vi "shared memory read.vi"(6 "channel classification":T1, 8 "error in":errorcluster, 10 "data table":T2, 11 "module in":refnum<class "Shared Memory Runtime.lvclass">) -> (0 "error out":errorcluster, 2 "data table out":T2, 3 "module out":refnum<class "Shared Memory Runtime.lvclass">)   [LabVIEW 2013, in "Shared Memory Runtime.lvclass"]
uses:
  Shared Memory Runtime.lvclass
  <vilib>/NI/Tag Bus/table/data table.ctl
  <vilib>/NI/Tag Bus Module Framework/channel/channel classification.ctl
  <vilib>/NI/Tag Bus/table/data polymorphs/write many/write Doubles.vi
  <vilib>/NI/Tag Bus/table/data polymorphs/write many/write Singles.vi
  <vilib>/NI/Tag Bus/table/data polymorphs/write many/write I64s.vi
  <vilib>/NI/Tag Bus/table/data polymorphs/write many/write I32s.vi
  <vilib>/NI/Tag Bus/table/data polymorphs/write many/write I16s.vi
  <vilib>/NI/Tag Bus/table/data polymorphs/write many/write I8s.vi
  <vilib>/NI/Tag Bus/table/data polymorphs/write many/write U64s.vi
  <vilib>/NI/Tag Bus/table/data polymorphs/write many/write U32s.vi
  <vilib>/NI/Tag Bus/table/data polymorphs/write many/write U16s.vi
  <vilib>/NI/Tag Bus/table/data polymorphs/write many/write U8s.vi
  <vilib>/NI/Tag Bus/table/data polymorphs/write many/write Booleans.vi
  <vilib>/National Instruments/Shared Memory Library for Linux RT/VIs/Miscellaneous/Get Shared Object Path.vi
  <vilib>/Utility/libraryn.llb/Check if File or Folder Exists.vi
  <vilib>/Utility/error.llb/Error Cluster From Error Code.vi
  <vilib>/NI/Tag Bus/table/data table.lvlib
  <vilib>/National Instruments/Shared Memory Library for Linux RT/Shared Memory.lvlib
  <vilib>/NI/Tag Bus Module Framework/channel/TBM channel.lvclass
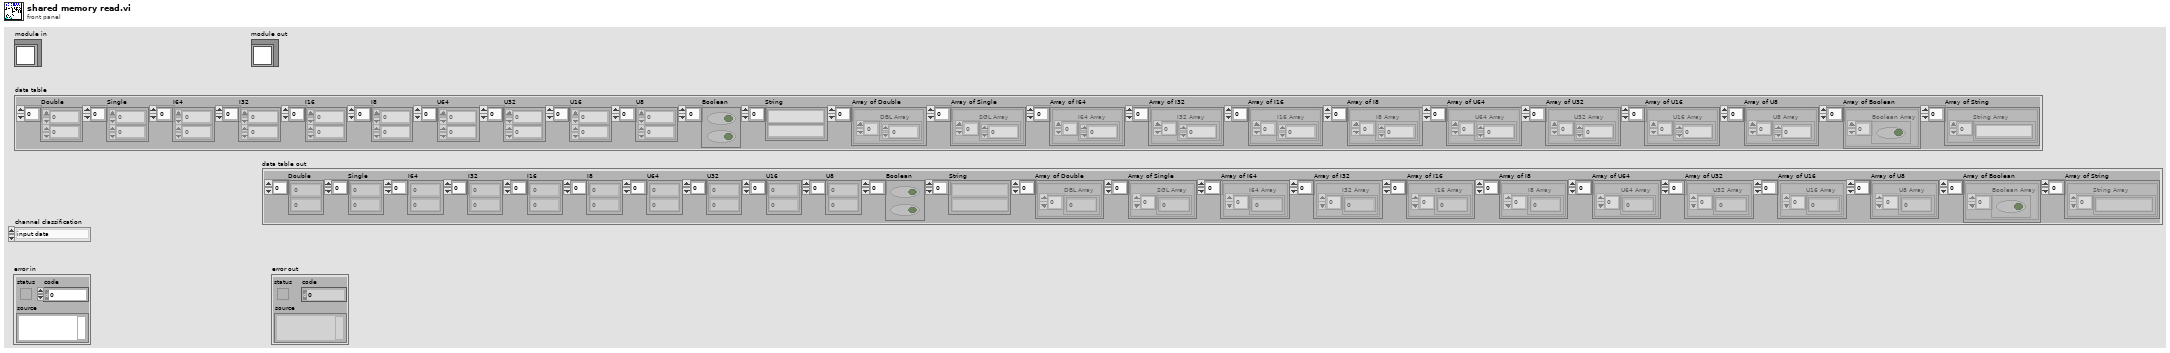
[diagram p1: front panel]
types:
  T1 = typedef "TBM channel.lvclass/channel classification.ctl" = enum16{"input data", "output data", "processing parameter", "processing result"}
  T2 = typedef "tag bus.lvlib/data table.lvlib/data table.ctl" = cluster{"Double":dbl[], "Single":sgl[], "I64":i64[], "I32":i32[], "I16":i16[], "I8":i8[], "U64":u64[], "U32":u32[], "U16":u16[], "U8":u8[], "Boolean":bool[], "String":string[], "Array of Double":cluster{"DBL Array":dbl[]}[], "Array of Single":cluster{"SGL Array":sgl[]}[], "Array of I64":cluster{"I64 Array":i64[]}[], "Array of I32":cluster{"I32 Array":i32[]}[], "Array of I16":cluster{"I16 Array":i16[]}[], "Array of I8":cluster{"I8 Array":i8[]}[], "Array of U64":cluster{"U64 Array":u64[]}[], "Array of U32":cluster{"U32 Array":u32[]}[], "Array of U16":cluster{"U16 Array":u16[]}[], "Array of U8":cluster{"U8 Array":u8[]}[], "Array of Boolean":cluster{"Boolean Array":bool[]}[], "Array of String":cluster{"String Array":string[]}[]}
  T3 = typedef "shared memory runtime.lvclass/shared memory module runtime.ctl" = cluster{"channel classification":T1, "data type":T4, "pointer to shared memory":u64, "number of elements":u64, "data dictionary index":cluster{i32[]}, "shared memory":T5}
  T4 = typedef "tag bus.lvlib/tag descriptor.lvclass/Data Type.ctl" = enum16{"Double", "Single", "I64", "I32", "I16", "I8", "U64", "U32", "U16", "U8", "Boolean", "String", "Array of Double", "Array of Single", "Array of I64", "Array of I32", "Array of I16", "Array of I8", "Array of U64", "Array of U32", "Array of U16", "Array of U8", "Array of Boolean", "Array of String"}
  T5 = typedef "Shared Memory Class Reference.ctl" = refnum<data-value>
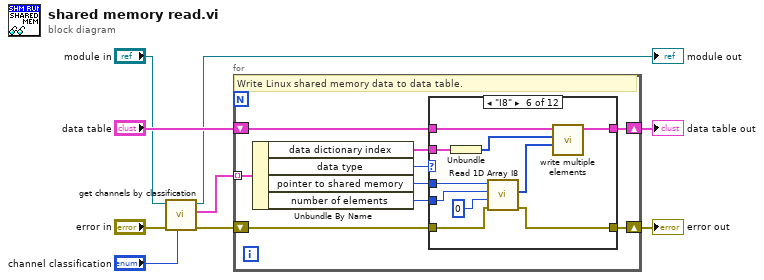
[diagram p0: block diagram]
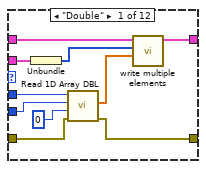
[diagram p2: hidden frame]
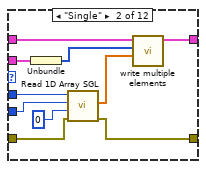
[diagram p3: hidden frame]
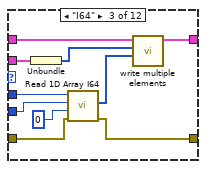
[diagram p4: hidden frame]
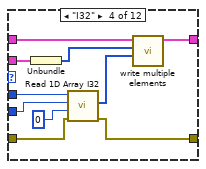
[diagram p5: hidden frame]
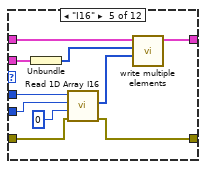
[diagram p6: hidden frame]
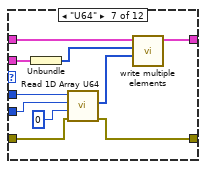
[diagram p7: hidden frame]
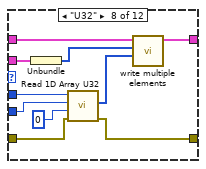
[diagram p8: hidden frame]
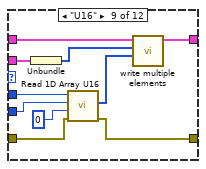
[diagram p9: hidden frame]
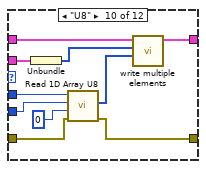
[diagram p10: hidden frame]
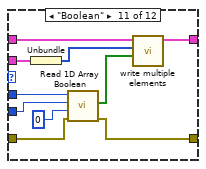
[diagram p11: hidden frame]
diagram:
  n1 = call "get channels by classification.vi"("channel classification"="channel classification", "error in"="error in", "shared memory runtime in"="module in") -> ("error out"=w1:errorcluster, "channels"=w4:T3[], "shared memory runtime out"=→"module out":refnum<class "Shared Memory Runtime.lvclass">)  [unwired: 6 in]
  n2 = for {
    tunnel: w4 -> [w16] mode=indexing
    shift-right: [w11] -> w7
    shift-left: w1 -> [w12]
    shift-right: [w18] -> w8
    shift-left: "data table" -> [w17]
    # "Write Linux shared memory data to data table."
    n3 = Unbundle By Name(w16) -> ("data dictionary index"=w10:cluster{i32[]}, "data type"=w13:T4, "pointer to shared memory"=w15:u64, "number of elements"=w14:u64)
    n4 = case shown="\"I8\"" w13 {
      tunnel: w17 -> [w28 w38 w48 w58 w68 w78 w88 w98 w108 w118 w128 w130]
      tunnel: [w27 w37 w47 w57 w67 w77 w87 w97 w107 w117 w127 w130] -> w18
      tunnel: w12 -> [w20 w30 w40 w50 w60 w70 w80 w90 w100 w110 w121 w129]
      tunnel: [w19 w29 w39 w49 w59 w69 w79 w89 w99 w109 w120 w129] -> w11
      tunnel: w15 -> [w22 w32 w42 w52 w62 w72 w82 w92 w102 w112 w123 _]
      tunnel: w14 -> [w21 w31 w41 w51 w61 w71 w81 w91 w101 w111 w122 _]
      tunnel: w10 -> [w26 w36 w46 w56 w66 w76 w86 w96 w106 w116 w126 _]
      frame "Double" {
        n5 = Unbundle(w26) -> (w25:i32[])
        n6 = call <vilib>:"Read 1D Array DBL.vi"("error in (no error)"=w20, "start index"=u64 0, "number of elements"=w21, "pointer"=w22) -> ("error out"=w19:errorcluster, "value"=w23:dbl[])  [unwired: 5 in, 1 out]
        n7 = call-poly <vilib>:"write multiple elements.vi"("values"=w23, "indices"=w25, "data table in"=w28) -> ("data table out"=w27:T2)  [unwired: 8 in]
      }
      frame "Single" {
        n8 = Unbundle(w36) -> (w35:i32[])
        n9 = call <vilib>:"Read 1D Array SGL.vi"("error in (no error)"=w30, "start index"=u64 0, "number of elements"=w31, "pointer"=w32) -> ("error out"=w29:errorcluster, "value"=w33:sgl[])  [unwired: 5 in, 1 out]
        n10 = call-poly <vilib>:"write multiple elements.vi"("values"=w33, "indices"=w35, "data table in"=w38) -> ("data table out"=w37:T2)  [unwired: 8 in]
      }
      frame "I64" {
        n11 = Unbundle(w46) -> (w45:i32[])
        n12 = call <vilib>:"Read 1D Array I64.vi"("error in (no error)"=w40, "start index"=u64 0, "number of elements"=w41, "pointer"=w42) -> ("error out"=w39:errorcluster, "value"=w43:i64[])  [unwired: 5 in, 1 out]
        n13 = call-poly <vilib>:"write multiple elements.vi"("values"=w43, "indices"=w45, "data table in"=w48) -> ("data table out"=w47:T2)  [unwired: 8 in]
      }
      frame "I32" {
        n14 = Unbundle(w56) -> (w55:i32[])
        n15 = call <vilib>:"Read 1D Array I32.vi"("error in (no error)"=w50, "start index"=u64 0, "number of elements"=w51, "pointer"=w52) -> ("error out"=w49:errorcluster, "value"=w53:i32[])  [unwired: 5 in, 1 out]
        n16 = call-poly <vilib>:"write multiple elements.vi"("values"=w53, "indices"=w55, "data table in"=w58) -> ("data table out"=w57:T2)  [unwired: 8 in]
      }
      frame "I16" {
        n17 = Unbundle(w66) -> (w65:i32[])
        n18 = call <vilib>:"Read 1D Array I16.vi"("error in (no error)"=w60, "start index"=u64 0, "number of elements"=w61, "pointer"=w62) -> ("error out"=w59:errorcluster, "value"=w63:i16[])  [unwired: 5 in, 1 out]
        n19 = call-poly <vilib>:"write multiple elements.vi"("values"=w63, "indices"=w65, "data table in"=w68) -> ("data table out"=w67:T2)  [unwired: 8 in]
      }
      frame "I8" {
        n20 = Unbundle(w76) -> (w75:i32[])
        n21 = call <vilib>:"Read 1D Array I8.vi"("error in (no error)"=w70, "start index"=u64 0, "number of elements"=w71, "pointer"=w72) -> ("error out"=w69:errorcluster, "value"=w73:i8[])  [unwired: 5 in, 1 out]
        n22 = call-poly <vilib>:"write multiple elements.vi"("values"=w73, "indices"=w75, "data table in"=w78) -> ("data table out"=w77:T2)  [unwired: 8 in]
      }
      frame "U64" {
        n23 = Unbundle(w86) -> (w85:i32[])
        n24 = call <vilib>:"Read 1D Array U64.vi"("error in (no error)"=w80, "start index"=u64 0, "number of elements"=w81, "pointer"=w82) -> ("error out"=w79:errorcluster, "value"=w83:u64[])  [unwired: 5 in, 1 out]
        n25 = call-poly <vilib>:"write multiple elements.vi"("values"=w83, "indices"=w85, "data table in"=w88) -> ("data table out"=w87:T2)  [unwired: 8 in]
      }
      frame "U32" {
        n26 = Unbundle(w96) -> (w95:i32[])
        n27 = call <vilib>:"Read 1D Array U32.vi"("error in (no error)"=w90, "start index"=u64 0, "number of elements"=w91, "pointer"=w92) -> ("error out"=w89:errorcluster, "value"=w93:u32[])  [unwired: 5 in, 1 out]
        n28 = call-poly <vilib>:"write multiple elements.vi"("values"=w93, "indices"=w95, "data table in"=w98) -> ("data table out"=w97:T2)  [unwired: 8 in]
      }
      frame "U16" {
        n29 = Unbundle(w106) -> (w105:i32[])
        n30 = call <vilib>:"Read 1D Array U16.vi"("error in (no error)"=w100, "start index"=u64 0, "number of elements"=w101, "pointer"=w102) -> ("error out"=w99:errorcluster, "value"=w103:u16[])  [unwired: 5 in, 1 out]
        n31 = call-poly <vilib>:"write multiple elements.vi"("values"=w103, "indices"=w105, "data table in"=w108) -> ("data table out"=w107:T2)  [unwired: 8 in]
      }
      frame "U8" {
        n32 = Unbundle(w116) -> (w115:i32[])
        n33 = call <vilib>:"Read 1D Array U8.vi"("error in (no error)"=w110, "start index"=u64 0, "number of elements"=w111, "pointer"=w112) -> ("error out"=w109:errorcluster, "value"=w113:u8[])  [unwired: 5 in, 1 out]
        n34 = call-poly <vilib>:"write multiple elements.vi"("values"=w113, "indices"=w115, "data table in"=w118) -> ("data table out"=w117:T2)  [unwired: 8 in]
      }
      frame "Boolean" {
        n35 = Unbundle(w126) -> (w125:i32[])
        n36 = call <vilib>:"Read 1D Array Boolean.vi"("error in (no error)"=w121, "start index"=u64 0, "number of elements"=w122, "pointer"=w123) -> ("error out"=w120:errorcluster, "value"=w119:bool[])  [unwired: 5 in, 1 out]
        n37 = call-poly <vilib>:"write multiple elements.vi"("values"=w119, "indices"=w125, "data table in"=w128) -> ("data table out"=w127:T2)  [unwired: 8 in]
      }
      frame Default {
      }
    }
  }
  "error out" <- w7
  "data table out" <- w8
